vi "Write NCh 1Samp (DBL).vi"(5 "timestamp":timestamp, 7 "index_channel":u32, 8 "error in":errorcluster, 9 "data":dbl[](array[numeric]), 10 "channels":u32[](array[numeric]), 11 "Writer":refnum<class "Synnax Writer.lvclass">) -> (0 "error out":errorcluster, 3 "Writer Out":refnum<class "Synnax Writer.lvclass">)   [LabVIEW 2026, in "synnax_clib.lvlib" / "Synnax Writer.lvclass"]
uses:
  Synnax Writer.lvclass
  Synnax Writer.lvclass/Synnax Writer.ctl
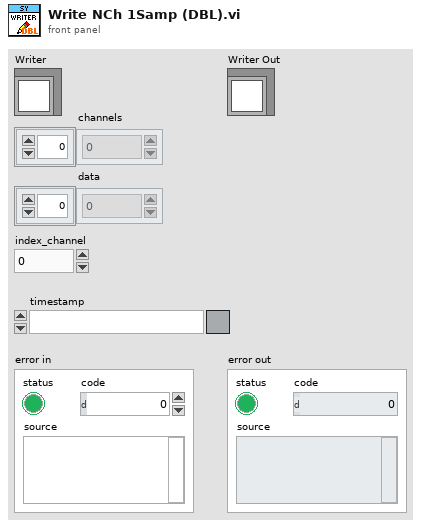
[diagram p1: front panel]
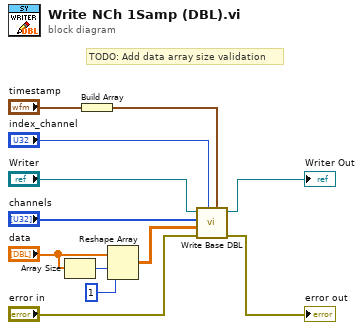
[diagram p0: block diagram]
diagram:
  # "TODO: Add data array size validation"
  n1 = Array Size(array="data") -> (size(s)=w4:i32)
  n2 = Build Array("timestamp") -> (w8:timestamp[])
  n3 = Reshape Array("data", w4, 1) -> (w6:dbl[][])
  n4 = call "Write Base DBL.vi"("timestamps"=w8, "index_channel"="index_channel", "error in"="error in", "data"=w6, "channels"="channels", "Writer"="Writer") -> ("error out"=→"error out":errorcluster, "Writer Out"=→"Writer Out":refnum<class "Synnax Writer.lvclass">)  [unwired: 4 in]
